vi "MGCC_PlannedISD_main.vi"   [LabVIEW 2016]
uses:
  Finite State Machine/Sub-VIs/MGCC_FntStaMach_gobal.vi
  Model Management/Global_MdlMgmt.vi
  <vilib>/imath/engines/lvmath2/RunTimeEngine/IndexRead/NIMS M($,S).vi
  <instcachedir>/0/NIMS M($,S)_3E5749BBB62E49528D4765A77F1F6D98.lvgen/NIMS M($,S)_3E5749BBB62E49528D4765A77F1F6D98_000.vi
  <vilib>/imath/engines/lvmath2/RunTimeEngine/BuiltInFunctions/length/NIMS_length(GV).vi
  <instcachedir>/0/NIMS_length(GV)_08A3D13377FD4E4B96F5795FBF3698FA.lvgen/NIMS_length(GV)_08A3D13377FD4E4B96F5795FBF3698FA_000.vi
  <vilib>/imathl/engines/lvmath/Functions/Error Handling/Create Error.vi
  <vilib>/imath/engines/lvmath2/RunTimeEngine/RangeToken/NIMS_Range_R3 - Integer.vi
  <instcachedir>/0/NIMS_Range_R3 - Integer_A435E2FF893B4C718FD5055FE39FE2F6.lvgen/NIMS_Range_R3 - Integer_A435E2FF893B4C718FD5055FE39FE2F6_000.vi
  <vilib>/imath/engines/lvmath2/RunTimeEngine/CommandStatement/MC_CommandStatement_break.vi
  <vilib>/imath/engines/lvmath2/RunTimeEngine/IndexRead/NIMS M(S,S).vi
  <instcachedir>/0/NIMS M(S,S)_AC51E74150A542F7991B9634C66F3096.lvgen/NIMS M(S,S)_AC51E74150A542F7991B9634C66F3096_000.vi
  <vilib>/imath/engines/lvmath2/RunTimeEngine/RowToken/NIMS_RowToken_M_SorRV.vi
  <instcachedir>/0/NIMS_RowToken_M_SorRV_4D710C5E6F8040F3A39B2F03436798DB.lvgen/NIMS_RowToken_M_SorRV_4D710C5E6F8040F3A39B2F03436798DB_002.vi
  <vilib>/imath/engines/lvmath2/RunTimeEngine/ErrorHandling/NIMS_Create Error From Enums.vi
  <vilib>/imath/engines/lvmath2/RunTimeEngine/BuiltInFunctions/sort/NIMS_[1o]_sort(RM,I32,Str).vi
  <instcachedir>/0/NIMS_[1o]_sort(RM,I32,Str)_6AE83B8BDD0442B0B72A0445EEE0CEB4.lvgen/NIMS_[1o]_sort(RM,I32,Str)_6AE83B8BDD0442B0B72A0445EEE0CEB4_000.vi
  <vilib>/imath/engines/lvmath2/RunTimeEngine/BuiltInFunctions/length/NIMS_length(GM).vi
  <instcachedir>/0/NIMS_length(GM)_47CEC356FCE0482D9BA47DC61C99F2C7.lvgen/NIMS_length(GM)_47CEC356FCE0482D9BA47DC61C99F2C7_000.vi
  <vilib>/imath/engines/lvmath2/RunTimeEngine/IndexRead/NIMS M(S).vi
  <instcachedir>/0/NIMS M(S)_B826C018497E4940AE96BD27B540B6FB.lvgen/NIMS M(S)_B826C018497E4940AE96BD27B540B6FB_000.vi
  <vilib>/imath/engines/lvmath2/RunTimeEngine/BuiltInFunctions/findnz/NIMS_[1o]_findnz(GRowV).vi
  <instcachedir>/0/NIMS_[1o]_findnz(GRowV)_1AF74843B4874134ADE908C0A4A72F3C.lvgen/NIMS_[1o]_findnz(GRowV)_1AF74843B4874134ADE908C0A4A72F3C_000.vi
  <vilib>/imath/engines/lvmath2/RunTimeEngine/BuiltInFunctions/is_empty/NIMS_is_empty(GV).vi
  <instcachedir>/0/NIMS_is_empty(GV)_FC7E7C3D9544432CB6AA2416ADCF6D56.lvgen/NIMS_is_empty(GV)_FC7E7C3D9544432CB6AA2416ADCF6D56_000.vi
  <vilib>/imath/engines/lvmath2/RunTimeEngine/BuiltInFunctions/findnz/NIMS_[1o]_findnz(GM).vi
  <instcachedir>/0/NIMS_[1o]_findnz(GM)_0B85F0C1FD7A4D70A7D15487030BA0C8.lvgen/NIMS_[1o]_findnz(GM)_0B85F0C1FD7A4D70A7D15487030BA0C8_003.vi
  <vilib>/imath/engines/lvmath2/RunTimeEngine/BuiltInFunctions/is_empty/NIMS_is_empty(GM).vi
  <instcachedir>/0/NIMS_is_empty(GM)_AF8F13F4B7FD436CB1855477E2504B8A.lvgen/NIMS_is_empty(GM)_AF8F13F4B7FD436CB1855477E2504B8A_005.vi
  <vilib>/imath/engines/lvmath2/RunTimeEngine/IndexRead/NIMS M(S,$).vi
  <instcachedir>/0/NIMS M(S,$)_F24F360562DE41D8BE234322A2E15C65.lvgen/NIMS M(S,$)_F24F360562DE41D8BE234322A2E15C65_000.vi
  <vilib>/imath/engines/lvmath2/RunTimeEngine/NodeEndStatement/NIMS_NodeEndStatement_Output.vi
  <instcachedir>/0/NIMS_NodeEndStatement_Output_53EC0D466D134D7ABD903AC30B43404B.lvgen/NIMS_NodeEndStatement_Output_53EC0D466D134D7ABD903AC30B43404B_005.vi
  <vilib>/imath/engines/lvmath2/RunTimeEngine/ErrorHandling/NIMS_Finalize Error.vi
  Communication/Global communication.vi
  <vilib>/imath/engines/lvmath2/RunTimeEngine/Managers/WorkSpace/UID Generator.vi
  <vilib>/imath/engines/lvmath2/RunTimeEngine/IndexReplace/NIMS V(S)=S.vi
  <instcachedir>/0/NIMS V(S)=S_57E16554CB8B4B90AAB163894F717546.lvgen/NIMS V(S)=S_57E16554CB8B4B90AAB163894F717546_000.vi
  <vilib>/imath/engines/lvmath2/RunTimeEngine/BuiltInFunctions/findnz/NIMS_[1o]_findnz(GColV).vi
  <instcachedir>/0/NIMS_[1o]_findnz(GColV)_8556557C9365446B906472366DD9B2D8.lvgen/NIMS_[1o]_findnz(GColV)_8556557C9365446B906472366DD9B2D8_000.vi
  <instcachedir>/0/NIMS_length(GV)_08A3D13377FD4E4B96F5795FBF3698FA.lvgen/NIMS_length(GV)_08A3D13377FD4E4B96F5795FBF3698FA_002.vi
  <vilib>/imath/engines/lvmath2/RunTimeEngine/BuiltInFunctions/zeros/NIMS_M=zeros(I32,I32).vi
  <vilib>/imath/engines/lvmath2/RunTimeEngine/RangeToken/NIMS_Range_R2 - Integer.vi
  <instcachedir>/0/NIMS_Range_R2 - Integer_89B873E74E6E489885E44F751DD9C6BF.lvgen/NIMS_Range_R2 - Integer_89B873E74E6E489885E44F751DD9C6BF_000.vi
  <vilib>/imath/engines/lvmath2/RunTimeEngine/IndexRead/NIMS V(S).vi
  <instcachedir>/0/NIMS V(S)_0488751826AF41519A22953C041130DC.lvgen/NIMS V(S)_0488751826AF41519A22953C041130DC_000.vi
  <instcachedir>/0/NIMS V(S)_0488751826AF41519A22953C041130DC.lvgen/NIMS V(S)_0488751826AF41519A22953C041130DC_002.vi
  <vilib>/imath/engines/lvmath2/RunTimeEngine/IndexReplace/NIMS M(S,S)=S.vi
  <instcachedir>/0/NIMS M(S,S)=S_98E40400474E4398B113AE20298B4F82.lvgen/NIMS M(S,S)=S_98E40400474E4398B113AE20298B4F82_002.vi
  <vilib>/imath/engines/lvmath2/RunTimeEngine/ArithmeticOperatorToken/NIMS_ArithmeticOperator_times.vi
  <instcachedir>/0/NIMS_ArithmeticOperator_times_953B34F74CAC448FB707D816A29CC5F0.lvgen/NIMS_ArithmeticOperator_times_953B34F74CAC448FB707D816A29CC5F0_000.vi
  <vilib>/imath/engines/lvmath2/RunTimeEngine/ArithmeticOperatorToken/NIMS_ArithmeticOperator_multmx(M,CV).vi
  <instcachedir>/0/NIMS_ArithmeticOperator_multmx(M,CV)_EE734FC8520844C9A7CC1A67008668A3.lvgen/NIMS_ArithmeticOperator_multmx(M,CV)_EE734FC8520844C9A7CC1A67008668A3_001.vi
  <vilib>/imath/engines/lvmath2/RunTimeEngine/RunTimeType/NIMS_RunTimeType_From StrictType (excl LVString).vi
  <instcachedir>/0/NIMS_RunTimeType_From StrictType (excl LVString)_BBF44FB49F834B71AF7A14CCEDF8BECD.lvgen/NIMS_RunTimeType_From StrictType (excl LVString)_BBF44FB49F834B71AF7A14CCEDF8BECD_000.vi
  <vilib>/imath/engines/lvmath2/RunTimeEngine/RunTimeType/NIMS_RunTimeType_Set Source Original Bool.vi
  <vilib>/imath/engines/lvmath2/RunTimeEngine/LocalVariableDefStatement/MC_LocalVariableDefStatement_Display.vi
  <vilib>/imath/engines/lvmath2/RunTimeEngine/IndexReplace/NIMS M(S)=S.vi
  <instcachedir>/0/NIMS M(S)=S_B3274CDAFA9346529812A4A947D623CC.lvgen/NIMS M(S)=S_B3274CDAFA9346529812A4A947D623CC_001.vi
  <vilib>/imath/engines/lvmath2/RunTimeEngine/Managers/SymbolTable/Clear UID.vi
  <instcachedir>/0/NIMS_NodeEndStatement_Output_53EC0D466D134D7ABD903AC30B43404B.lvgen/NIMS_NodeEndStatement_Output_53EC0D466D134D7ABD903AC30B43404B_001.vi
  <instcachedir>/0/NIMS_NodeEndStatement_Output_53EC0D466D134D7ABD903AC30B43404B.lvgen/NIMS_NodeEndStatement_Output_53EC0D466D134D7ABD903AC30B43404B_002.vi
  Communication/Global communication output.vi
  <vilib>/imath/engines/lvmath2/RunTimeEngine/Managers/SymbolTable/NIMS_WorkSpace.lvlib
panel:
  # "Copyright <2020> <The University of Tennessee at Knoxville and the University of Tennessee Research Foundation>\n\nRedistribution and use in source and binary forms, with or without modification, are permitted provided that the following conditions are met:\n\n1. Redistributions of source code must retain the above copyright notice, this list of conditions and the following disclaimer.\n\n2. Redistributions in binary form must reproduce the above copyright notice, this list of conditions and the following disclaimer in the documentation and/or other materials provided with the distribution.\n\n3. Neither the name of the copyright holder nor the names of its contributors may be used to endorse or promote products derived from this software without specific prior written permission.\n\nTHIS SOFTWARE IS PROVIDED BY THE COPYRIGHT HOLDERS AND CONTRIBUTORS \"AS IS\" AND ANY EXPRESS OR IMPLIED WARRANTIES, INCLUDING, BUT NOT LIMITED TO, THE IMPLIED WARRANTIES OF MERCHANTABILITY AND FITNESS FOR A PARTICULAR PURPOSE ARE DISCLAIMED. IN NO EVENT SHALL THE COPYRIGHT HOLDER OR CONTRIBUTORS BE LIABLE FOR ANY DIRECT, INDIRECT, INCIDENTAL, SPECIAL, EXEMPLARY, OR CONSEQUENTIAL DAMAGES (INCLUDING, BUT NOT LIMITED TO, PROCUREMENT OF SUBSTITUTE GOODS OR SERVICES; LOSS OF USE, DATA, OR PROFITS; OR BUSINESS INTERRUPTION) HOWEVER CAUSED AND ON ANY THEORY OF LIABILITY, WHETHER IN CONTRACT, STRICT LIABILITY, OR TORT (INCLUDING NEGLIGENCE OR OTHERWISE) ARISING IN ANY WAY OUT OF THE USE OF THIS SOFTWARE, EVEN IF ADVISED OF THE POSSIBILITY OF SUCH DAMAGE."
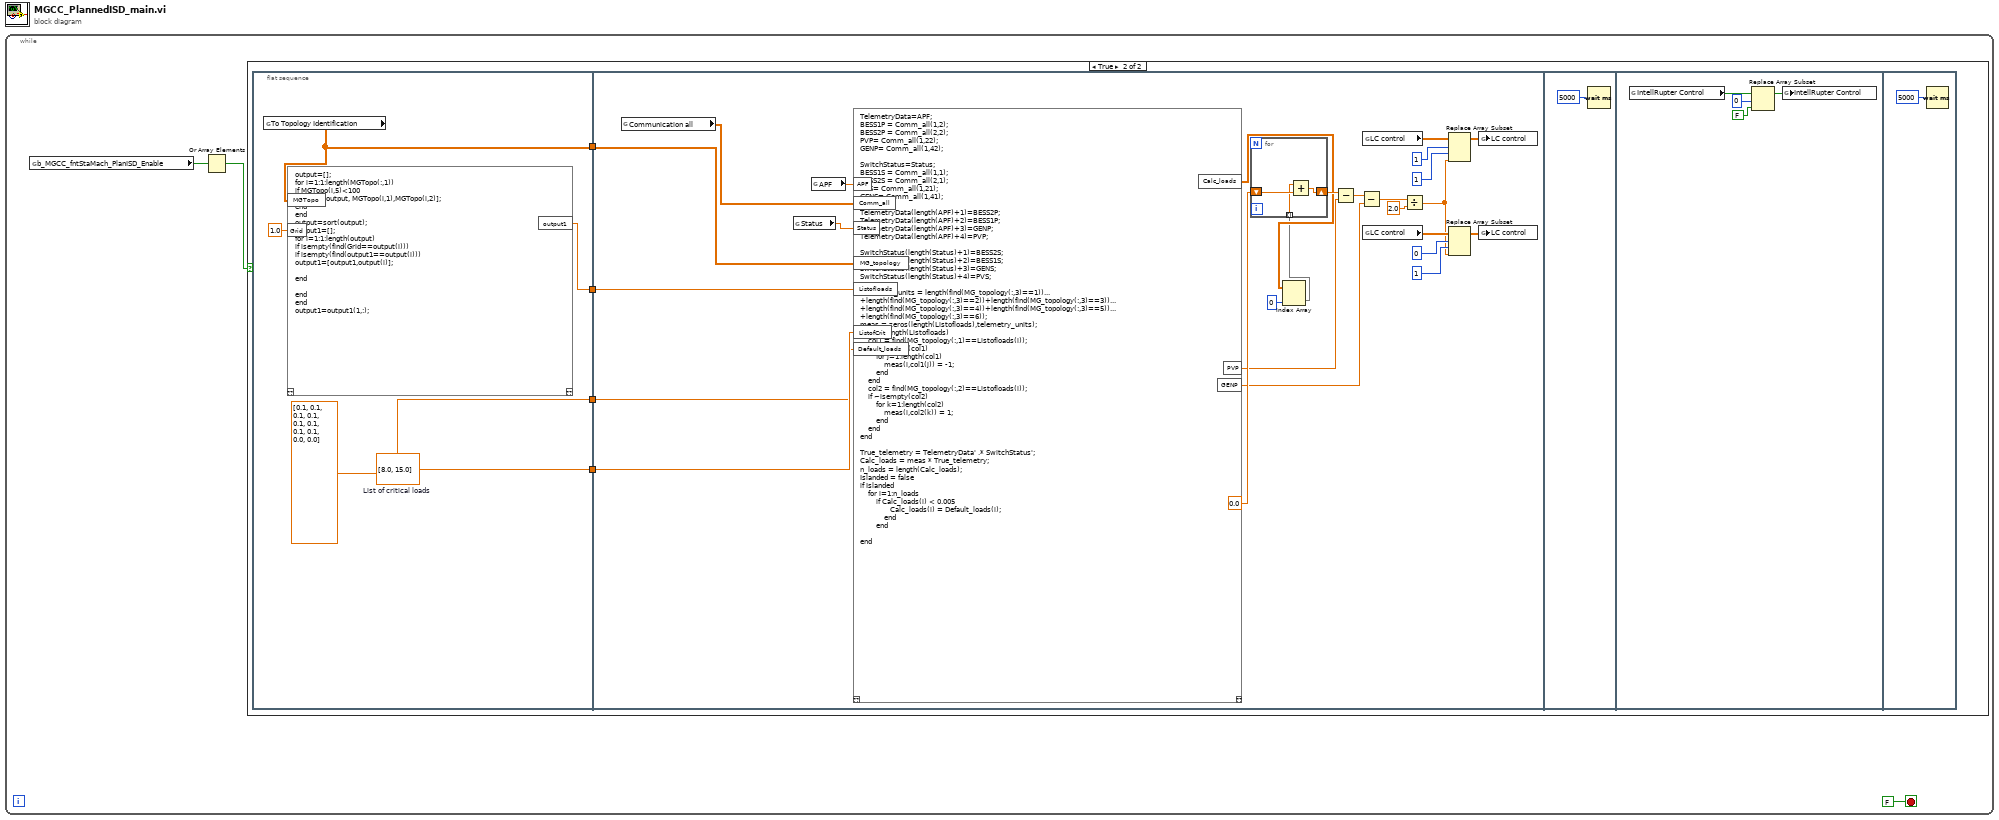
[diagram p0: block diagram]
diagram:
  n1 = while {
    stop <- FALSE stop-if-true
    n2 = global read "MGCC_FntStaMach_gobal.vi" "b_MGCC_fntStaMach_PlanISD_Enable"() -> (w3:bool[])
    n3 = Or Array Elements(Boolean array=w3) -> (logical OR=w1:bool)
    n4 = case shown="True" w1 {
      frame False {
      }
      frame True {
        n5 = flat-sequence {
          tunnel: [w11] -> w7
          tunnel: [w10] -> w6
          tunnel: [w9] -> w5
          tunnel: [dbl[] [0.1, 0.1, 0.1, 0.1, 0.1, 0.1, 0.1, 0.1, 0.0, 0.0]] -> w4
          tunnel: w7 -> [w333]
          tunnel: w6 -> [w331]
          tunnel: w5 -> [w330]
          tunnel: w4 -> [w329]
          frame #0 {
            w9 = dbl[] [8.0, 15.0]  # List of critical loads
            n6 = global read "Global_MdlMgmt.vi" "To Topology Identification"() -> (w10:dbl[][])
            n7 = mathscript code="output=[];\nfor i=1:1:length(MGTopo(:,1))\nif MGTopo(i,5)<100\noutput=[output, MGTopo(i,1),MGTopo(i,2)];\nend\nend\noutput=sort(output);\noutput1=[];\nfor i=1:1:length(output)\nif isempty(find(Grid==output(i)))\nif isempty(find(output1==output(i)))\noutput1=[output1,output(i)];\n\nend\n\nend\nend\noutput1=output1(1,:);"("MGTopo"=w10, "Grid"=1.0) -> ("output1"=w11:dbl[])  [unwired: 1 in, 1 out]
          }
          frame #1 {
            n8 = global read "Global communication.vi" "Communication all"() -> (w332:dbl[][])
            n9 = global read "Global communication.vi" "Status"() -> (w334:dbl[])
            n10 = global read "Global communication.vi" "APF"() -> (w349:dbl[])
            n11 = mathscript code="TelemetryData=APF;\nBESS1P = Comm_all(1,2);\nBESS2P = Comm_all(2,2);\nPVP= Comm_all(1,22);\nGENP= Comm_all(1,42);\n\nSwitchStatus=Status;\nBESS1S = Comm_all(1,1);\nBESS2S = Comm_all(2,1);\nPVS= Comm_all(1,21);\nGENS= Comm_all(1,41);\n\nTelemetryData(length(APF)+1)=BESS2P;\nTelemetryData(length(APF)+2)=BESS1P;\nTelemetryData(length(APF)+3)=GENP;\nTelemetryData(length(APF)+4)=PVP;\n\nSwitchStatus(length(Status)+1)=BESS2S;\nSwitchStatus(length(Status)+2)=BESS1S;\nSwitchStatus(length(Status)+3)=GENS;\nSwitchStatus(length(Status)+4)=PVS;\n\ntelemetry_units = length(find(MG_topology(:,3)==1))...\n+length(find(MG_topology(:,3)==2))+length(find(MG_topology(:,3)==3))...\n+length(find(MG_topology(:,3)==4))+length(find(MG_topology(:,3)==5))...\n+length(find(MG_topology(:,3)==6));\nmeas = zeros(length(Listofloads),telemetry_units);\nfor i=1:length(Listofloads)\n    col1 = find(MG_topology(:,1)==Listofloads(i));\n    if ~isempty(col1)\n        for j=1:length(col1)\n            meas(i,col1(j)) = -1;\n        end\n    end\n    col2 = find(MG_topology(:,2)==Listofloads(i));\n    if ~isempty(col2)\n        for k=1:length(col2)\n            meas(i,col2(k)) = 1;\n        end\n    end\nend\n\nTrue_telemetry = TelemetryData' .* SwitchStatus';\nCalc_loads = meas * True_telemetry;\nn_loads = length(Calc_loads);\nIslanded = false\nif Islanded\n    for i=1:n_loads\n        if Calc_loads(i) < 0.005\n               Calc_loads(i) = Default_loads(i);\n            end\n        end\n\nend"("APF"=w349, "Comm_all"=w332, "Status"=w334, "Listofloads"=w333, "MG_topology"=w331, "ListofCrit"=w330, "Default_loads"=w329) -> ("Calc_loads"=w327:dbl[][], "PVP"=w325:dbl, "GENP"=w324:dbl)  [unwired: 1 in, 1 out]
            n12 = Index Array(array=w327, index (col)=0 ("disabled index (col)")) -> (element=w326:dbl[])  [unwired: 1 in]
            n13 = for {
              shift-right: [w351] -> w347
              shift-left: 0.0 -> [w352]
              tunnel: w326 -> [w350] mode=indexing
              n14 = Add(x=w350, y=w352) -> (x+y=w351:dbl)
            }
            n15 = Subtract(x=w347, y=w325) -> (x-y=w346:dbl)
            n16 = Subtract(x=w346, y=w324) -> (x-y=w345:dbl)
            n17 = global read "Global communication.vi" "LC control"() -> (w339:dbl[][])
            n18 = global read "Global communication.vi" "LC control"() -> (w342:dbl[][])
            n19 = Divide(x=w345, y=2.0) -> (x/y=w335:dbl)
            n20 = Replace Array Subset(array=w339, new element=w335, index (row)=1 ("index"), index (col)=1 ("index")) -> (w338:dbl[][])
            n21 = Replace Array Subset(array=w342, new element=w335, index (row)=0 ("index"), index (col)=1 ("index")) -> (w343:dbl[][])
            n22 = global write "Global communication.vi" "LC control"(w338) -> ()
            n23 = global write "Global communication.vi" "LC control"(w343) -> ()
          }
          frame #2 {
            n24 = Wait (ms)(milliseconds to wait=u32 5000) -> ()  [unwired: 1 out]
          }
          frame #3 {
            n25 = global read "Global communication output.vi" "IntellRupter Control"() -> (w1318:bool[])
            n26 = Replace Array Subset(array=w1318, new element=FALSE ("new element/subarray"), index=0) -> (w1315:bool[])
            n27 = global write "Global communication output.vi" "IntellRupter Control"(w1315) -> ()
          }
          frame #4 {
            n28 = Wait (ms)(milliseconds to wait=u32 5000) -> ()  [unwired: 1 out]
          }
        }
      }
    }
  }
